vi "Example Simple.vi"() -> ()   [LabVIEW 2013]
uses:
  C:/tf/play/labview/Tinkerforge.dll
panel:
  out "voltage (V)":sgl
  out "current (A)":sgl
  in  "uid":string="amb"
  in  "port":i32=4223
  in  "host":string="localhost"
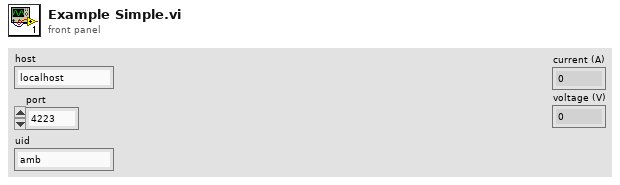
[diagram p1: front panel]
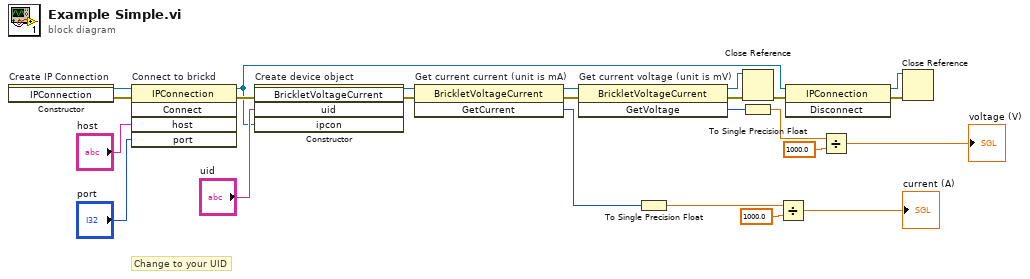
[diagram p0: block diagram]
diagram:
  # "Change to your UID"
  n1 = constructor on="Create IP Connection" class="IPConnection"() -> (reference out=w24:refnum<k24>, error out=w9:errorcluster)  [unwired: 3 in, 1 out]
  n2 = invoke on="Connect to brickd" class="IPConnection" method="Connect"(reference=w24, error in=w9, "host"="host", "port"="port") -> (reference out=w15:refnum<k24>, error out=w20:errorcluster)  [unwired: 1 in, 3 out]
  n3 = constructor on="Create device object" class="BrickletVoltageCurrent"(error in=w20, "uid"="uid", "ipcon"=w15) -> (reference out=w18:refnum<k24>, error out=w19:errorcluster)  [unwired: 2 in, 3 out]
  n4 = invoke on="Get current current (unit is mA)" class="BrickletVoltageCurrent" method="GetCurrent"(reference=w18, error in=w19) -> (reference out=w7:refnum<k24>, error out=w8:errorcluster, "GetCurrent"=w13:i32)  [unwired: 1 in]
  n5 = invoke on="Get current voltage (unit is mV)" class="BrickletVoltageCurrent" method="GetVoltage"(reference=w7, error in=w8) -> (reference out=w5:refnum<k24>, error out=w6:errorcluster, "GetVoltage"=w3:i32)  [unwired: 1 in]
  n6 = To Single Precision Float(number=w13) -> (single precision float=w11:sgl)
  n7 = Close Reference(reference=w5, error in (no error)=w6) -> (error out=w17:errorcluster)
  n8 = To Single Precision Float(number=w3) -> (single precision float=w1:sgl)
  n9 = Divide(x=w11, y=sgl 1000.0) -> (x/y=→"current (A)":sgl)
  n10 = invoke class="IPConnection" method="Disconnect"(reference=w15, error in=w17) -> (reference out=w14:refnum<k24>, error out=w16:errorcluster)  [unwired: 1 in, 1 out]
  n11 = Divide(x=w1, y=sgl 1000.0) -> (x/y=→"voltage (V)":sgl)
  n12 = Close Reference(reference=w14, error in (no error)=w16) -> ()  [unwired: 1 out]
